vi "Draw Speaker.vi"(0 "picture in":picture, 5 "center":cluster{"X":i32, "Y":i32}, 7 "width":i32, 9 "state":T1, 11 "active":bool) -> (4 "picture out":picture)   [LabVIEW 2020, in "SAC Config.xctl"]
uses:
  SAC Config.xctl
  Speaker State.ctl
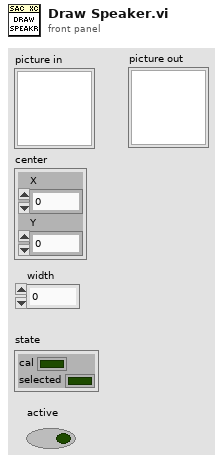
[diagram p1: front panel]
types:
  T1 = typedef "SAC Config.xctl/Speaker State.ctl" = cluster{"cal":bool, "selected":bool}
  T2 = cluster{"Width":u16, "Style":enum32{"Solid", "Dash", "Dot", "DashDot", "DashDotDot"}}
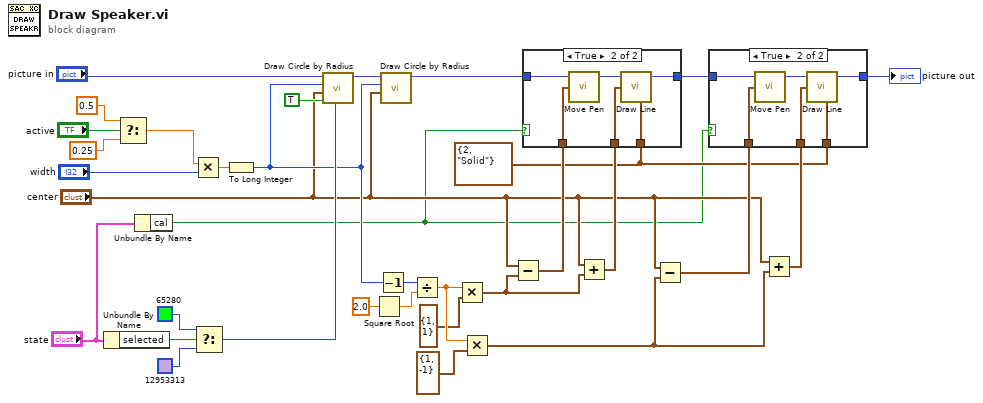
[diagram p0: block diagram]
diagram:
  w3 = T2 {"Width"=2, "Style"=enum."Solid"} ("pen")
  n1 = Unbundle By Name("state") -> ("selected"=w24:bool)
  n2 = Select(t=0.5, s="active", f=0.25) -> (s? t:f=w26:dbl)
  n3 = Unbundle By Name("state") -> ("cal"=w1:bool)
  n4 = Multiply(x=w26, y="width") -> (x*y=w29:dbl)
  n5 = Select(t=u32 65280 ("color(black)"), s=w24, f=u32 12953313 ("color(black)")) -> (s? t:f=w21:u32)
  n6 = To Long Integer(number=w29) -> (32bit integer=w20:i32)
  n7 = call <vilib>:"Draw Circle by Radius.vi"("color(black)"=w21, "fill?(F)"=TRUE, "pixel center"="center", "radius"=w20, "picture"="picture in") -> ("new picture"=w33:picture)  [unwired: 6 in]
  n8 = Square Root(x=2.0) -> (sqrt(x)=w18:dbl)
  n9 = Decrement(x=w20) -> (x-1=w19:i32)
  n10 = call <vilib>:"Draw Circle by Radius.vi"("pixel center"="center", "radius"=w20, "picture"=w33) -> ("new picture"=w16:picture)  [unwired: 8 in]
  n11 = Divide(x=w19, y=w18) -> (x/y=w14:dbl)
  n12 = Multiply(x=w14, y=cluster{"x":i16, "y":i16} {"x"=1, "y"=1} ("new position")) -> (x*y=w11:cluster{"x":dbl, "y":dbl})
  n13 = Multiply(x=w14, y=cluster{"x":i16, "y":i16} {"x"=1, "y"=-1} ("new position")) -> (x*y=w6:cluster{"x":dbl, "y":dbl})
  n14 = Subtract(x="center", y=w11) -> (x-y=w12:cluster{dbl, dbl})
  n15 = Add(x="center", y=w11) -> (x+y=w10:cluster{dbl, dbl})
  n16 = case shown="True" w1 {
    tunnel: w16 -> [w34 w40]
    tunnel: w12 -> [_ w39]
    tunnel: w10 -> [_ w37]
    tunnel: [w34 w36] -> w9
    tunnel: w3 -> [_ w35]
    frame False {
    }
    frame True {
      n17 = call <vilib>:"Move Pen.vi"("new position"=w39, "picture"=w40) -> ("new picture"=w38:picture)  [unwired: 3 in]
      n18 = call <vilib>:"Draw Line.vi"("picture"=w38, "end point"=w37, "pen"=w35) -> ("new picture"=w36:picture)  [unwired: 6 in]
    }
  }
  n19 = Subtract(x="center", y=w6) -> (x-y=w8:cluster{dbl, dbl})
  n20 = Add(x="center", y=w6) -> (x+y=w5:cluster{dbl, dbl})
  n21 = case shown="True" w1 {
    tunnel: w9 -> [w41 w47]
    tunnel: w8 -> [_ w46]
    tunnel: w5 -> [_ w44]
    tunnel: [w41 w43] -> w4
    tunnel: w3 -> [_ w42]
    frame False {
    }
    frame True {
      n22 = call <vilib>:"Move Pen.vi"("new position"=w46, "picture"=w47) -> ("new picture"=w45:picture)  [unwired: 3 in]
      n23 = call <vilib>:"Draw Line.vi"("picture"=w45, "end point"=w44, "pen"=w42) -> ("new picture"=w43:picture)  [unwired: 6 in]
    }
  }
  "picture out" <- w4
